vi "FpgaSession_GET.vi"(8 "error in":errorcluster, 11 "lia host in":refnum<class "LIA Host Interface FPGA.lvclass">) -> (0 "error out":errorcluster, 2 "fpga session out":refnum<k20>, 3 "lia host out":refnum<class "LIA Host Interface FPGA.lvclass">)   [LabVIEW 2017, in "LIA Host Interface FPGA.lvclass"]
uses:
  LIA Host Interface FPGA.lvclass
  LIA Host Interface FPGA.lvclass/LIA Host Interface FPGA.ctl
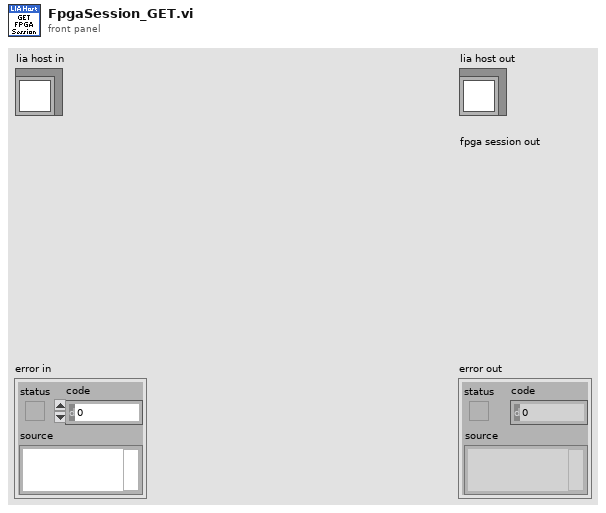
[diagram p1: front panel]
types:
  T1 = typedef "LIA Host Interface Desktop.lvclass/session data.ctl" = cluster{"fpga session":refnum<k20>, "record length":u32[]}
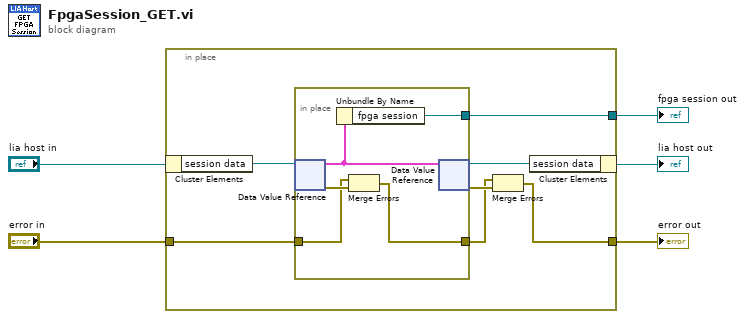
[diagram p0: block diagram]
diagram:
  n1 = in-place {
    in-place-border: [w10] -> w1
    in-place-border: "error in" -> [w9]
    in-place-border: [w6] -> w2
    n2 = in-place-cluster #1("lia host in") -> ("session data"=w12:refnum<data-value>)
    n3 = in-place {
      in-place-border: [w16] -> w10
      in-place-border: w9 -> [w14]
      in-place-border: [w13] -> w7
      n4 = in-place-dvr #2(w12) -> (w17:T1, w15:errorcluster)
      n5 = Unbundle By Name(w17) -> ("fpga session"=w16:refnum<k20>)
      n6 = Merge Errors(w14, w15) -> (w13:errorcluster)
      n7 = in-place-dvr #2(w17) -> (w11:refnum<data-value>, w8:errorcluster)
    }
    n8 = Merge Errors(w7, w8) -> (w6:errorcluster)
    n9 = in-place-cluster #1("session data"=w11) -> (→"lia host out":refnum<class "LIA Host Interface FPGA.lvclass">)
  }
  "error out" <- w2
  "fpga session out" <- w1
